vi "Lecture5exercise2.vi"() -> ()   [LabVIEW 2022 SP3]
uses:
  <vilib>/sound2/lvsound2.llb/Sampling Mode.ctl
  <vilib>/Analysis/2dsp.llb/Real FFT.vi
  <vilib>/Analysis/2dsp.llb/Inverse Real FFT.vi
  <vilib>/sound2/lvsound2.llb/Sound Input Read (DBL).vi
  <vilib>/Analysis/NI_AALPro.lvlib
panel:
  in  "Cutoff Frequency":dbl
  out "Filtered":dbl[](graph)
  out "Filtered Spectrum":dbl[](graph)
  out "Spectrum":dbl[](graph)
  out "Original":dbl[](graph)
  in  "stop":bool
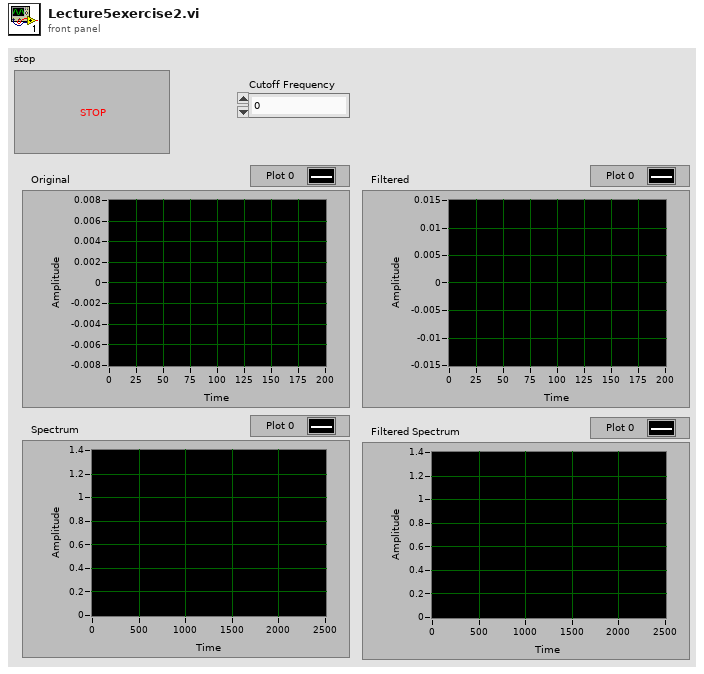
[diagram p1: front panel]
types:
  T1 = typedef "Sampling Mode.ctl" = i32
  T2 = typedef "Sound Input Task ID.ctl" = u32
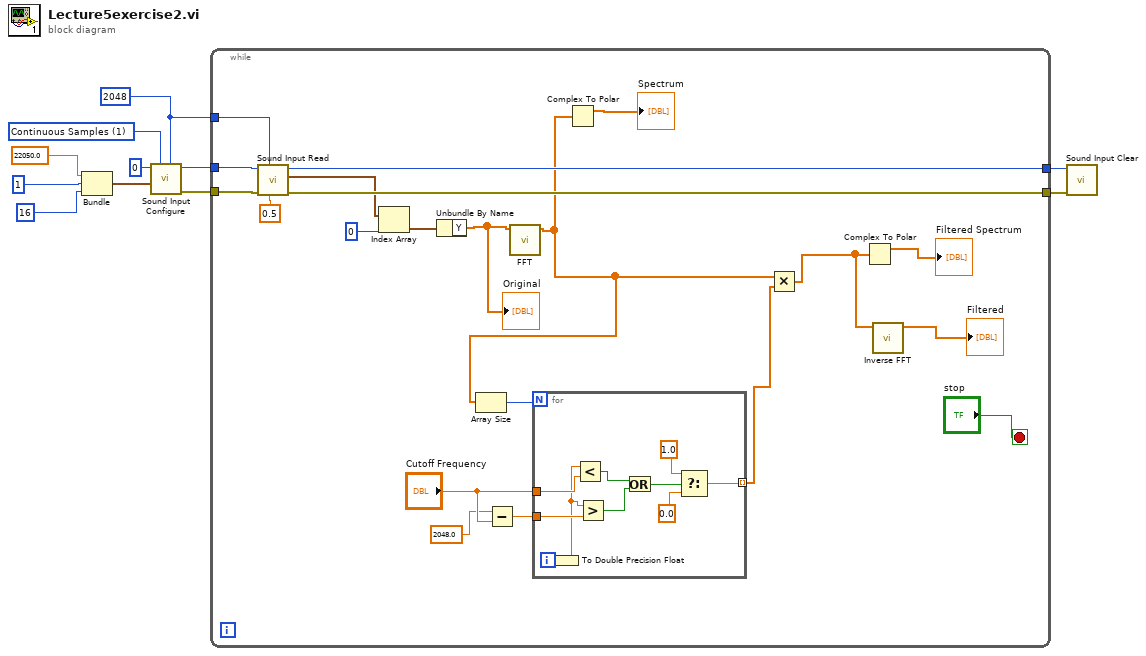
[diagram p0: block diagram]
diagram:
  w3 = 2048 ("number of samples/ch")
  w6 = T1 1 items=["Finite Samples", "Continuous Samples"] ("sample mode")
  n1 = Bundle(22050.0, 1, 16) -> (w8:cluster{dbl, i32, i32})  [unwired: 1 in]
  n2 = call <vilib>:"Sound Input Configure.vi"("number of samples/ch"=w3, "sample mode"=w6, "sound format"=w8, "device ID"=u32 0) -> ("error out"=w5:errorcluster, "task ID"=w4:T2)  [unwired: 6 in]
  n3 = while {
    tunnel: w5 -> [w28]
    tunnel: w4 -> [w27]
    tunnel: w3 -> [w26]
    tunnel: [w25] -> w2
    tunnel: [w24] -> w1
    stop <- "stop" stop-if-true
    n4 = call-poly <vilib>:"Sound Input Read.vi"("timeout (sec)"=0.5, "number of samples/ch"=w26, "error in (no error)"=w28, "task ID"=w27) -> ("error out"=w24:errorcluster, "data"=w23:waveform(dbl)[], "task ID out"=w25:T2)  [unwired: 5 in]
    n5 = Index Array(array=w23, index=0) -> (element=w29:waveform(dbl))
    n6 = Unbundle By Name(w29) -> ("Y"=w22:dbl[])
    "Original" <- w22
    n7 = Subtract(x=2048.0, y="Cutoff Frequency") -> (x-y=w14:dbl)
    n8 = call-poly <vilib>:"FFT.vi"("X"=w22) -> ("FFT {X}"=w12:cdb[])  [unwired: 9 in, 1 out]
    n9 = Array Size(array=w12) -> (size(s)=w13:i32)
    n10 = for {
      N: w13 -> [_]
      tunnel: [w40] -> w19 mode=indexing
      tunnel: "Cutoff Frequency" -> [w37]
      tunnel: w14 -> [w36]
      i -> [w35]
      n11 = To Double Precision Float(number=w35) -> (double precision float=w33:dbl)
      n12 = Less?(x=w33, y=w37) -> (x < y?=w38:bool)
      n13 = Greater?(x=w33, y=w36) -> (0:w34:bool)
      n14 = Or(x=w38, y=w34) -> (x .or. y?=w39:bool)
      n15 = Select(t=1.0, s=w39, f=0.0) -> (s? t:f=w40:dbl)
    }
    n16 = Complex To Polar(r * e^(i*theta)=w12) -> (r=→"Spectrum":dbl[])  [unwired: 1 out]
    n17 = Multiply(x=w12, y=w19) -> (x*y=w17:cdb[])
    n18 = Complex To Polar(r * e^(i*theta)=w17) -> (r=→"Filtered Spectrum":dbl[])  [unwired: 1 out]
    n19 = call-poly <vilib>:"Inverse FFT.vi"("FFT {X}"=w17) -> ("X"=→"Filtered":dbl[])  [unwired: 9 in, 1 out]
  }
  n20 = call <vilib>:"Sound Input Clear.vi"("error in (no error)"=w1, "task ID"=w2) -> ()  [unwired: 9 in, 1 out]
